vi "PrepareShutdownNotifier.vi"() -> (0 "error out":errorcluster, 3 "Notifier out":refnum<notifier>)   [LabVIEW 2013]
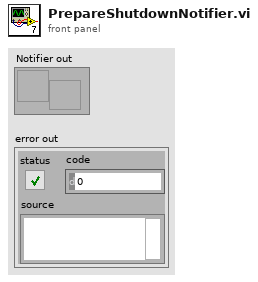
[diagram p1: front panel]
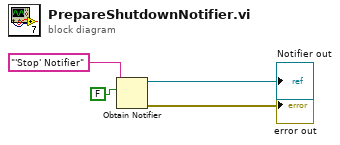
[diagram p0: block diagram]
diagram:
  n1 = Obtain Notifier(name (unnamed)="'Stop' Notifier", notification data type=FALSE) -> (notifier out=→"Notifier out":refnum<notifier>, error out=→"error out":errorcluster)  [unwired: 2 in, 1 out]
